vi "Read Message.vi"(8 "error in (no error)":errorcluster, 11 "Channel in":refnum<class "Channel.lvclass">) -> (0 "error out":errorcluster, 2 "Rx Message":string, 3 "Channel out":refnum<class "Channel.lvclass">)   [LabVIEW 2018, in "Channel.lvclass"]
uses:
  Channel.lvclass
  Channel.lvclass/Channel.ctl
  RxTx/RxTx.lvclass
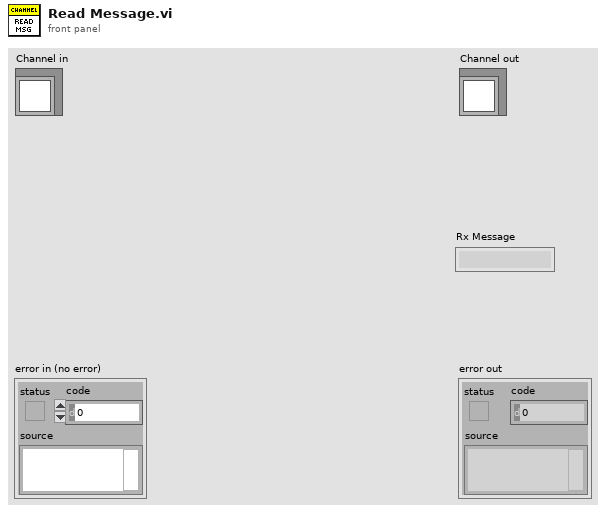
[diagram p1: front panel]
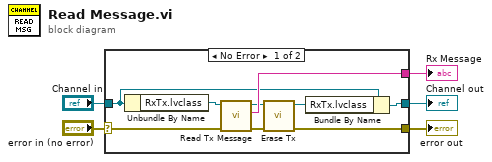
[diagram p0: block diagram]
diagram:
  n1 = case shown="No Error" "error in (no error)" {
    selector: "error in (no error)" -> [w13 w16]
    tunnel: [w6 w16] -> w4
    tunnel: [w8 w15] -> w2
    tunnel: "Channel in" -> [w9 w15]
    tunnel: [w12 _] -> w1
    frame No Error {
      n2 = Unbundle By Name(w9) -> ("RxTx.lvclass"=w14:refnum<class "RxTx.lvclass">)
      n3 = call "Read Tx Message.vi"("error in (no error)"=w13, "RxTx in"=w14) -> ("error out"=w11:errorcluster, "Tx Message"=w12:string, "RxTx out"=w10:refnum<class "RxTx.lvclass">)  [unwired: 7 in]
      n4 = call "Erase Tx.vi"("error in (no error)"=w11, "RxTx in"=w10) -> ("error out"=w6:errorcluster, "RxTx out"=w7:refnum<class "RxTx.lvclass">)  [unwired: 8 in]
      n5 = Bundle By Name(cluster=w9, "RxTx.lvclass"=w7) -> (w8:refnum<class "Channel.lvclass">)
    }
    frame Error {
    }
  }
  "error out" <- w4
  "Channel out" <- w2
  "Rx Message" <- w1
